vi "Convert and Enqueue.vi"(8 "error in":errorcluster, 11 "Data":u8[](array[numeric])) -> (0 "error out":errorcluster, 3 "Table Data":string[][](array[string]))   [LabVIEW 2025, in "Automotive Ethernet Bus Monitor UI.lvlib"]
doc: "Convert the recieved GetData payload and enqueue in the Table Queue"
uses:
  Automotive Ethernet Bus Monitor UI.lvlib
  Enqueue Data.vi
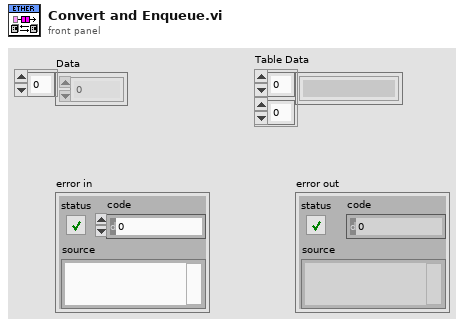
[diagram p1: front panel]
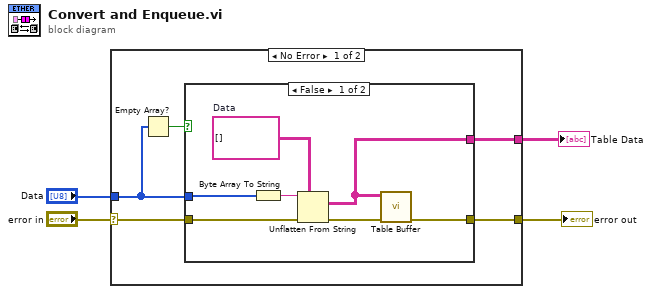
[diagram p0: block diagram]
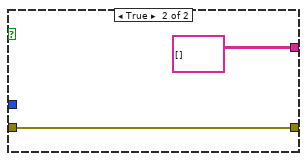
[diagram p2: hidden frame]
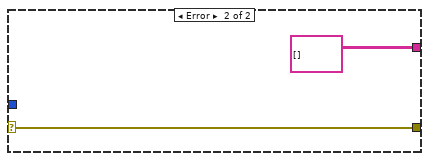
[diagram p3: hidden frame]
diagram:
  n1 = case shown="No Error" "error in" {
    selector: "error in" -> [w9 w20]
    tunnel: [w8 w20] -> w3
    tunnel: "Data" -> [w6 _]
    tunnel: [w5 string[][] [] ("Fetched I2C Messages")] -> w1
    frame No Error {
      n2 = Empty Array?(array=w6) -> (empty?=w7:bool)
      n3 = case shown="False" w7 {
        tunnel: w9 -> [w14 w18]
        tunnel: [w12 w18] -> w8
        tunnel: w6 -> [w16 _]
        tunnel: [w10 string[][] [] ("Fetched I2C Messages")] -> w5
        frame False {
          w13 = string[][] []  # Data
          n4 = Byte Array To String(unsigned byte array=w16) -> (string=w15:string)
          n5 = Unflatten From String(type=w13, binary string=w15, error in (no error)=w14) -> (value=w10:string[][], error out=w11:errorcluster)  [unwired: 2 in, 1 out]
          n6 = call-poly "Table Buffer.vi"("error in"=w11, "Data"=w10) -> ("error out"=w12:errorcluster)  [unwired: 8 in, 1 out]
        }
        frame True {
        }
      }
    }
    frame Error {
    }
  }
  "error out" <- w3
  "Table Data" <- w1
